vi "Read channel.vi"(8 "error in (no error)":errorcluster, 11 "OSAchannel in":refnum<class "OSAchannel.lvclass">) -> (0 "error out":errorcluster, 2 "channel":T1, 3 "OSAchannel out":refnum<class "OSAchannel.lvclass">)   [LabVIEW 2010, in "OSAchannel.lvclass"]
uses:
  OSAchannel.lvclass
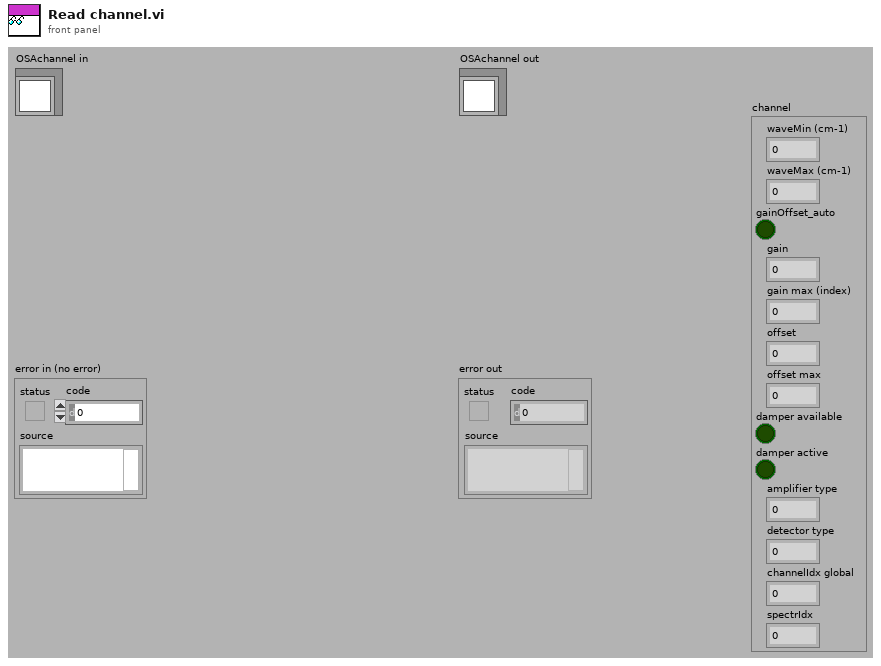
[diagram p1: front panel]
types:
  T1 = cluster{"waveMin (cm-1)":sgl, "waveMax (cm-1)":sgl, "gainOffset_auto":bool, "gain":i32, "gain max (index)":i32, "offset":i32, "offset max":i32, "damper available":bool, "damper active":bool, "amplifier type":i32, "detector type":i32, "channelIdx global":i32, "spectrIdx":u16}
  T2 = cluster{"waveMin (cm-1)":sgl, "waveMax (cm-1)":sgl, "gainOffset_auto":bool, "gain":i32, "gain levels nr":u16, "offset":i32, "offset max":u16, "damper available":bool, "damper active":bool, "amplifier type":i32, "detector type":i32, "channelIdx global":u16, "spectrIdx":u16, "waveMeter on":bool}
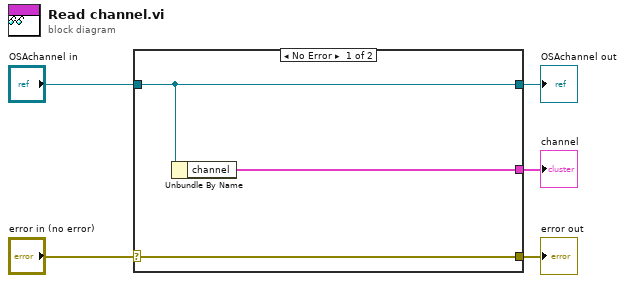
[diagram p0: block diagram]
diagram:
  n1 = case shown="No Error" "error in (no error)" {
    selector: "error in (no error)" -> [w8 w9]
    tunnel: [w8 w9] -> w4
    tunnel: [w7 w10] -> w2
    tunnel: "OSAchannel in" -> [w7 w10]
    tunnel: [w6 _] -> w1
    frame No Error {
      n2 = Unbundle By Name(w7) -> ("channel"=w6:T2)
    }
    frame Error {
    }
  }
  "error out" <- w4
  "OSAchannel out" <- w2
  "channel" <- w1
